vi "Add Mode Code Message-Subaddress Pair.vi"(4 "create timestamp channel":bool, 6 "parameters":T3(array[cluster]), 7 "mode code":u16=1, 8 "error in":errorcluster, 9 "terminals":cluster{"Rx":T4, "Tx":T4}, 10 "name":string, 11 "port":T1 format="%.0x") -> (0 "error out":errorcluster, 1 "message":T1 format="%.0x", 2 "subaddress":T1=18446744073709551615 format="%.0x", 3 "port out":T1 format="%.0x")   [LabVIEW 2020, in "AIM MIL-STD-1553 Scripting.lvlib"]
doc: "Adds a <b>mode code</b> to the Bus Controller as a <b>message</b> and adds a <b>subaddress</b> to the specified Remote Terminal from <b>terminals</b> (only RT->BC and BC-RT are supported)."
uses:
  AIM MIL-STD-1553 Scripting.lvlib
  <vilib>/NI VeriStand/Custom Device API/Custom Device Item Ref.ctl
  Shared/Terminal Endpoint.ctl
  Shared/Address.ctl
  Shared/Parameter Definition.ctl
  Shared/Message Type.ctl
  Constants.vi
  <vilib>/NI VeriStand/Custom Device API/Custom Device API.lvlib
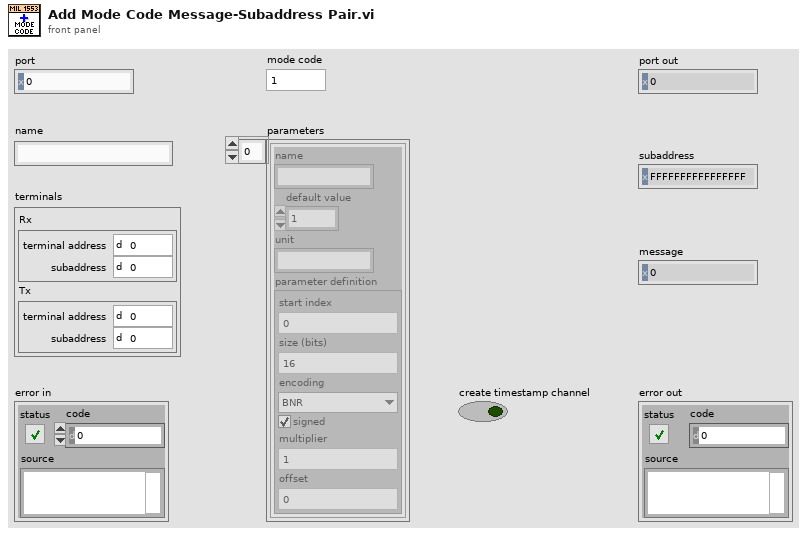
[diagram p1: front panel]
types:
  T1 = typedef "Custom Device API.lvlib/Custom Device Item Ref.ctl" = u64
  T2 = typedef "Parameter Definition.ctl" = cluster{"start index":i32, "size (bits)":i32, "encoding":enum16{"BNR", "BCD", "Discrete"}, "signed":bool, "multiplier":dbl, "offset":dbl}
  T3 = cluster{"name":string, "default value":dbl, "unit":string, "parameter definition":T2}[]
  T4 = typedef "Terminal Endpoint.ctl" = cluster{"terminal address":T5, "subaddress":T5}
  T5 = typedef "Address.ctl" = u16
  T6 = typedef "Message Type.ctl" = string
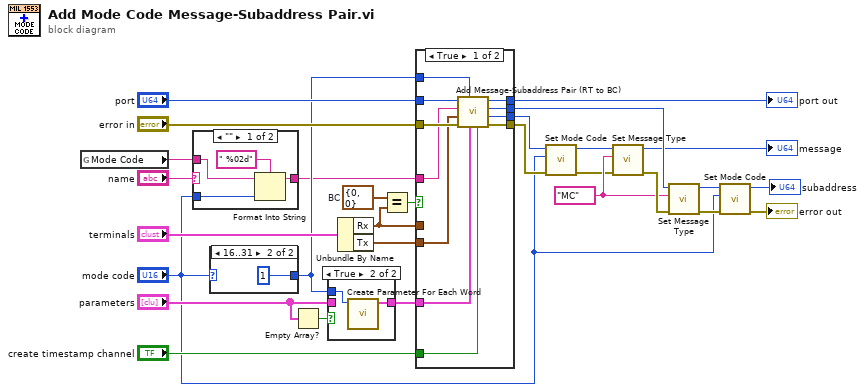
[diagram p0: block diagram]
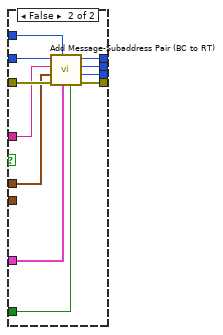
[diagram p3: hidden frame]
diagram:
  w12 = T6 "MC" ("message type")
  w26 = T4 {"terminal address"=0, "subaddress"=0}  # BC
  n1 = global read "Constants.vi" "Mode Code"() -> (w3:string)
  n2 = case shown="\"\"" "name" {
    selector: "name" -> [_ w34]
    tunnel: [w33 w34] -> w15
    tunnel: "mode code" -> [w32 _]
    tunnel: w3 -> [w30 _]
    frame "" {
      n3 = Format Into String(format string=" %02d", initial string=w30, w32) -> (resulting string=w33:string)  [unwired: 1 in, 1 out]
    }
    frame Default {
    }
  }
  n4 = case shown="16..31" "mode code" {
    tunnel: [_ u16 1 ("mode code")] -> w18
    frame Default {
    }
    frame 16..31 {
    }
  }
  n5 = Empty Array?(array="parameters") -> (empty?=w29:bool)
  n6 = case shown="True" w29 {
    tunnel: w18 -> [_ w38]
    tunnel: "parameters" -> [w36 _]
    tunnel: [w36 w37] -> w21
    frame False {
    }
    frame True {
      n7 = call "Create Parameter For Each Word.vi"("number of words"=w38) -> ("parameters"=w37:T3)  [unwired: 9 in, 1 out]
    }
  }
  n8 = Unbundle By Name("terminals") -> ("Rx"=w17:T4, "Tx"=w19:T4)
  n9 = Equal?(x=w26, y=w17) -> (x = y?=w25:bool)
  n10 = case shown="True" w25 {
    tunnel: "port" -> [w49 w60]
    tunnel: "error in" -> [w48 w59]
    tunnel: [w47 w58] -> w11
    tunnel: [w46 w57] -> w22
    tunnel: w21 -> [w45 w56]
    tunnel: "create timestamp channel" -> [w44 w55]
    tunnel: w15 -> [w43 w54]
    tunnel: w19 -> [w42 _]
    tunnel: w18 -> [w41 w53]
    tunnel: w17 -> [_ w52]
    tunnel: [w40 w51] -> w13
    tunnel: [w39 w50] -> w10
    frame True {
      n11 = call "Add Message-Subaddress Pair (RT to BC).vi"("create timestamp channel"=w44, "parameters"=w45, "number of words"=w41, "error in"=w48, "tx remote terminal"=w42, "name"=w43, "port"=w49) -> ("error out"=w47:errorcluster, "message"=w39:T1, "subaddress"=w40:T1, "port out"=w46:T1)  [unwired: 1 in]
    }
    frame False {
      n12 = call "Add Message-Subaddress Pair (BC to RT).vi"("create timestamp channel"=w55, "parameters"=w56, "number of words"=w53, "error in"=w59, "rx remote terminal"=w52, "name"=w54, "port"=w60) -> ("error out"=w58:errorcluster, "message"=w50:T1, "subaddress"=w51:T1, "port out"=w57:T1)  [unwired: 1 in]
    }
  }
  "port out" <- w22
  n13 = call "Set Mode Code.vi"("error in"=w11, "mode code"="mode code", "message or subaddress"=w10) -> ("error out"=w9:errorcluster, "message or subaddress out"=w8:T1)  [unwired: 7 in]
  n14 = call "Set Message Type.vi"("error in"=w9, "message type"=w12, "message or subaddress"=w8) -> ("error out"=w14:errorcluster, "message or subaddress out"=→"message":T1)  [unwired: 7 in]
  n15 = call "Set Message Type.vi"("error in"=w14, "message type"=w12, "message or subaddress"=w13) -> ("error out"=w6:errorcluster, "message or subaddress out"=w7:T1)  [unwired: 7 in]
  n16 = call "Set Mode Code.vi"("error in"=w6, "mode code"="mode code", "message or subaddress"=w7) -> ("error out"=→"error out":errorcluster, "message or subaddress out"=→"subaddress":T1)  [unwired: 7 in]
